vi "AutoSize Table Column with Header1.vi"() -> ()   [LabVIEW 2021]
panel:
  in  "Table":string[][](table)=[["aaaaaaaaaaa", "wer we qewrwer ", "wer ", "qwe r", "qwe rweqrwer", "were", "qwe rweqr "], ["a", "werwe", "", "", "", "", ""], ["aaaaaaaaaaaaaaaa", "", "", "", "asdf asd", "asd fsdf a", "dfa sdfasdfsdf asdf"]]
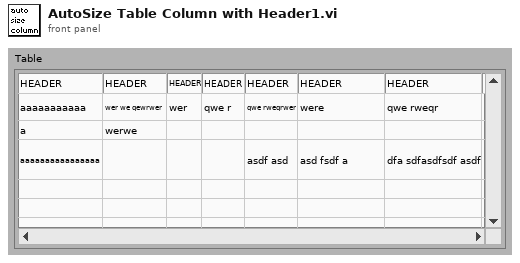
[diagram p1: front panel]
types:
  T1 = enum16{"User-specified Font", "Application Font", "System Font", "Dialog Font"}
  T2 = cluster{"Font Name:":string, "Size":i16, "Strikeout?":bool, "Italic?":bool, "Underline?":bool, "Outline?":bool, "Shadow?":bool, "Bold?":bool}
  T3 = cluster{"left":i16, "top":i16, "right":i16, "bottom":i16}
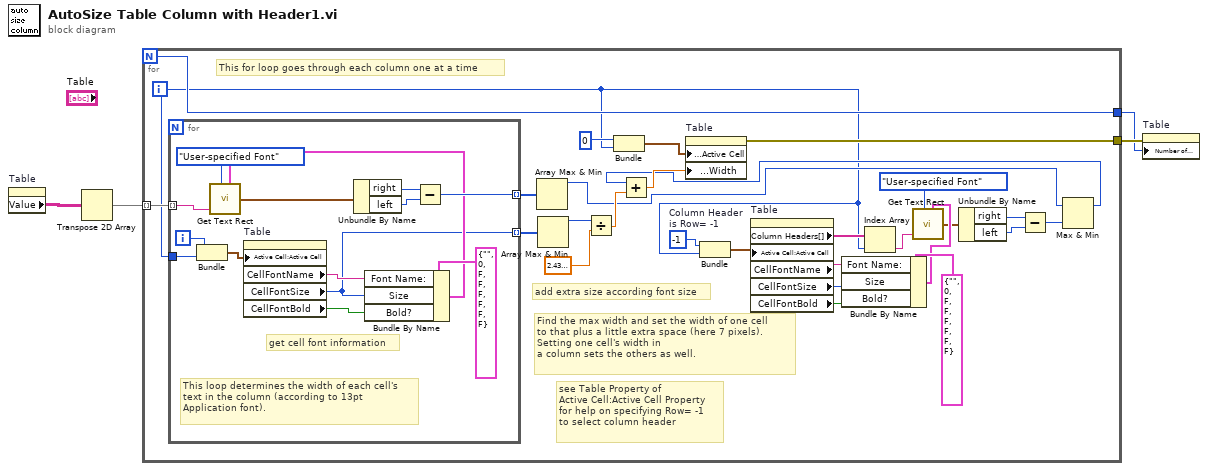
[diagram p0: block diagram]
diagram:
  n1 = property on="Table" class="Tbl (strict)"() -> ("Value"=w4:string[][])  [unwired: 2 in, 2 out]
  n2 = Transpose 2D Array(2D array=w4) -> (transposed array=w3:string[][])
  n3 = for {
    N -> [w22]
    tunnel: w3 -> [w32] mode=indexing
    tunnel: [w23] -> w2
    tunnel: [w22] -> w1
    i -> [w6]
    w5 = -1  # Column Header is Row= -1
    # "see Table Property of\nActive Cell:Active Cell Property\nfor help on specifying Row= -1\nto select column header"
    # "add extra size according font size"
    # "Find the max width and set the width of one cell \nto that plus a little extra space (here 7 pixels). \nSetting one cell's width in\na column sets the others as well."
    # "This for loop goes through each column one at a time"
    n4 = for {
      tunnel: w32 -> [w46] mode=indexing
      tunnel: [w42] -> w31 mode=indexing
      tunnel: w6 -> [w36]
      tunnel: [w33] -> w27 mode=indexing
      i -> [w35]
      # "get cell font information"
      # "This loop determines the width of each cell's\ntext in the column (according to 13pt\nApplication font)."
      n5 = Bundle(w35, w36) -> (w41:cluster{i32, i32})  [unwired: 1 in]
      n6 = property on="Table" class="Tbl (strict)"("Active Cell:Active Cell"=w41) -> ("CellFontName"=w40:string, "CellFontSize"=w33:u32, "CellFontBold"=w39:bool)  [unwired: 2 in, 2 out]
      n7 = Bundle By Name(cluster=T2 {"Font Name:"="", "Size"=0, "Strikeout?"=FALSE, "Italic?"=FALSE, "Underline?"=FALSE, "Outline?"=FALSE, "Shadow?"=FALSE, "Bold?"=FALSE} ("[user-specified font]"), "Font Name:"=w40, "Size"=w33, "Bold?"=w39) -> (w37:T2)
      n8 = call <vilib>:"Get Text Rect.vi"("desired font(Application)"=T1."User-specified Font", "text"=w46, "[user-specified font]"=w37) -> ("rect"=w45:T3)  [unwired: 6 in]
      n9 = Unbundle By Name(w45) -> ("right"=w44:i16, "left"=w43:i16)
      n10 = Subtract(x=w44, y=w43) -> (x-y=w42:i16)
    }
    n11 = Array Max & Min(array=w31) -> (max value=w8:i16)  [unwired: 3 out]
    n12 = Array Max & Min(array=w27) -> (max value=w26:u32)  [unwired: 3 out]
    n13 = Divide(x=w26, y=sgl 2.43) -> (x/y=w24:sgl)
    n14 = Bundle(0, w6) -> (w28:cluster{i32, i32})  [unwired: 1 in]
    n15 = Bundle("Column Header\nis Row= -1"=w5, w6) -> (w21:cluster{"Column Header\nis Row= -1":i32, i32})  [unwired: 1 in]
    n16 = property on="Table" class="Tbl (strict)"("Active Cell:Active Cell"=w21) -> ("Column Headers[]"=w20:string[], "CellFontName"=w19:string, "CellFontSize"=w18:u32, "CellFontBold"=w17:bool)  [unwired: 2 in, 2 out]
    n17 = Bundle By Name(cluster=T2 {"Font Name:"="", "Size"=0, "Strikeout?"=FALSE, "Italic?"=FALSE, "Underline?"=FALSE, "Outline?"=FALSE, "Shadow?"=FALSE, "Bold?"=FALSE} ("[user-specified font]"), "Font Name:"=w19, "Size"=w18, "Bold?"=w17) -> (w13:T2)
    n18 = Index Array(array=w20, index=w6) -> (element=w14:string)
    n19 = call <vilib>:"Get Text Rect.vi"("desired font(Application)"=T1."User-specified Font", "text"=w14, "[user-specified font]"=w13) -> ("rect"=w10:T3)  [unwired: 6 in]
    n20 = Unbundle By Name(w10) -> ("right"=w11:i16, "left"=w12:i16)
    n21 = Subtract(x=w11, y=w12) -> (x-y=w9:i16)
    n22 = Max & Min(x=w8, y=w9) -> (max(x,y)=w7:i16)  [unwired: 1 out]
    n23 = Add(x=w7, y=w24) -> (x+y=w29:sgl)
    n24 = property on="Table" class="Tbl (strict)"("Active Cell:Active Cell"=w28, "Active Cell:Cell Size:Width"=w29) -> (error out=w23:errorcluster)  [unwired: 2 in, 1 out]
  }
  n25 = property on="Table" class="Tbl (strict)"(error in=w2, "Number of Columns"=w1) -> ()  [unwired: 1 in, 2 out]
